vi "Read DI_index.vi"(11 "Heater in":refnum<class "Heater_v2.lvclass">) -> (2 "DI_index":i32, 3 "Heater out":refnum<class "Heater_v2.lvclass">)   [LabVIEW 2019, in "Heater_v2.lvclass"]
uses:
  Heater_v2.lvclass
  Heater_v2.lvclass/Heater_v2.ctl
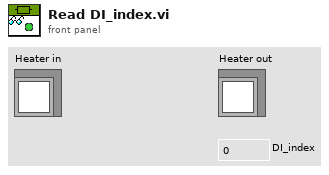
[diagram p1: front panel]
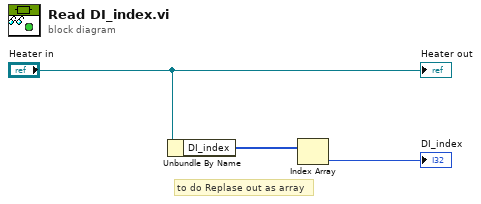
[diagram p0: block diagram]
diagram:
  # "to do Replase out as array"
  n1 = Unbundle By Name("Heater in") -> ("DI_index"=w1:i32[])
  n2 = Index Array(array=w1) -> (element=→"DI_index":i32)  [unwired: 1 in]
  "Heater out" <- "Heater in"
